vi "Programa funcion T co.vi"() -> ()   [LabVIEW 2020]
uses:
  <vilib>/addons/Control Design/_Model Construction/NI_LinSys_Model Creation.lvlib
  <vilib>/addons/Control Design/_Model Construction/NI_LinSys_Model Information.lvlib
  <vilib>/addons/Control Design/_Utility/NI_CD_Model Viewer.lvlib
  <vilib>/addons/Control Design/_Utility/Model Viewer.llb/Model Viewer SubVI/cd_Draw Transfer Function Equation (TF).vi
  <vilib>/addons/Control Design/_Model Construction/Model Information.llb/Model Information SubVIs/cd_Set Names To TF Model.vi
  <vilib>/addons/Control Design/_Model Construction/Model Creation.llb/Model Creation SubVI/cd_Create Transfer Function Model.vi
  <vilib>/functionblocks/Control/PID/PID.vi
  <vilib>/functionblocks/FB Core/FB Core.xnode
panel:
  out "?":T1(graph)={"Set-point (%)"=25.0, "Y% esc y filt"=25.0, "Ley uk"=12.500000564078626}
  in  "SET-POINT %":dbl
  in  "Ring":u16(ring) items=["LAZO ABIERTO", "LAZO CERRADO"]
  out "Y(k)":dbl
  out "X(t)":dbl[](array[numeric])
  in  "stop":bool
  in  "RETARDO":dbl
  in  "DENOMIDADOR":dbl[](array[numeric])
  in  "NUMERADOR":dbl[](array[numeric])
  out "Funcion de transferencia":picture
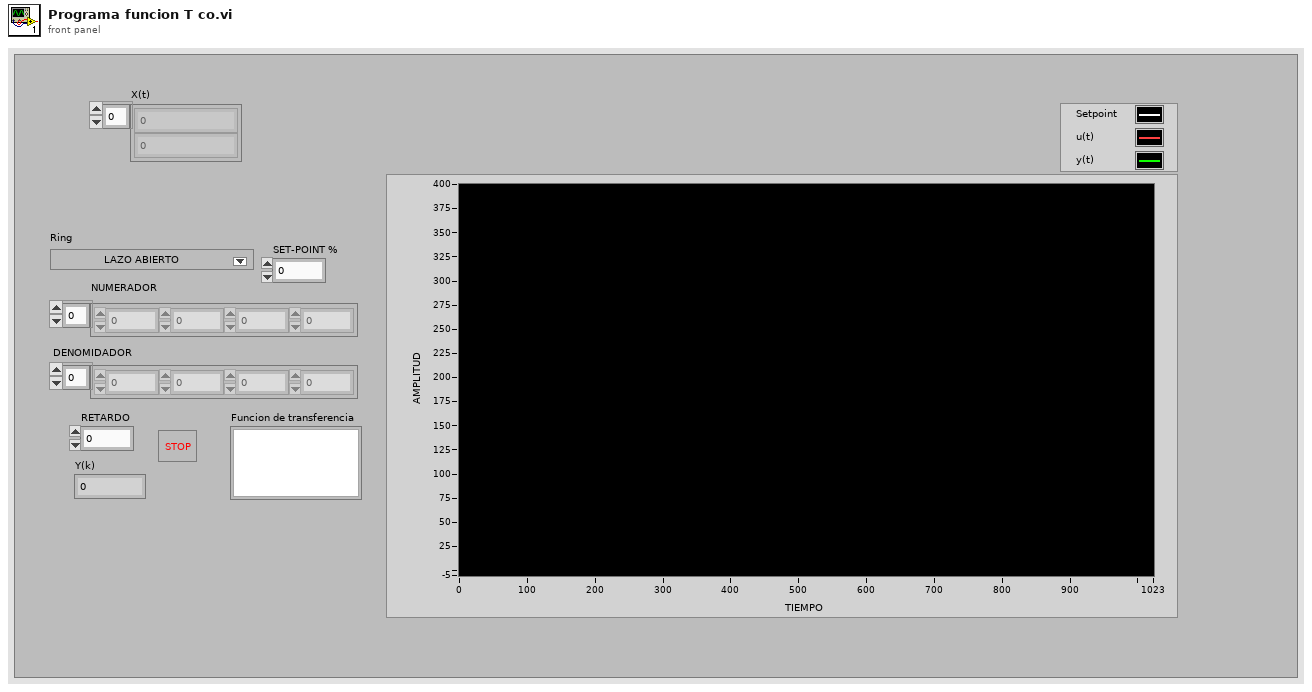
[diagram p1: front panel]
types:
  T1 = cluster{"Set-point (%)":dbl, "Y% esc y filt":dbl, "Ley uk":dbl}
  T2 = typedef "NI_Matrix.lvlib/RealMatrix.ctl" = dbl[][]
  T3 = cluster{"SET-POINT %":dbl, "output":dbl, "Y(k)":dbl}
  T4 = typedef "NI_LinSys_Model Typedefs.lvlib/CD Transfer Function Model (MIMO).ctl" = cluster{"properties":T5, "transfer function(s)":T6[][]}
  T5 = typedef "NI_LinSys_Model Typedefs.lvlib/CD General Elements.ctl" = cluster{"Model name":string, "Input names":string[], "Output names":string[], "Input Delays":dbl[], "Output Delays":dbl[], "Sampling Time":dbl, "Notes":string}
  T6 = typedef "NI_LinSys_Model Typedefs.lvlib/CD Transfer Function Model (SISO).ctl" = cluster{"Numerator":dbl[], "Denominator":dbl[], "delay":dbl}
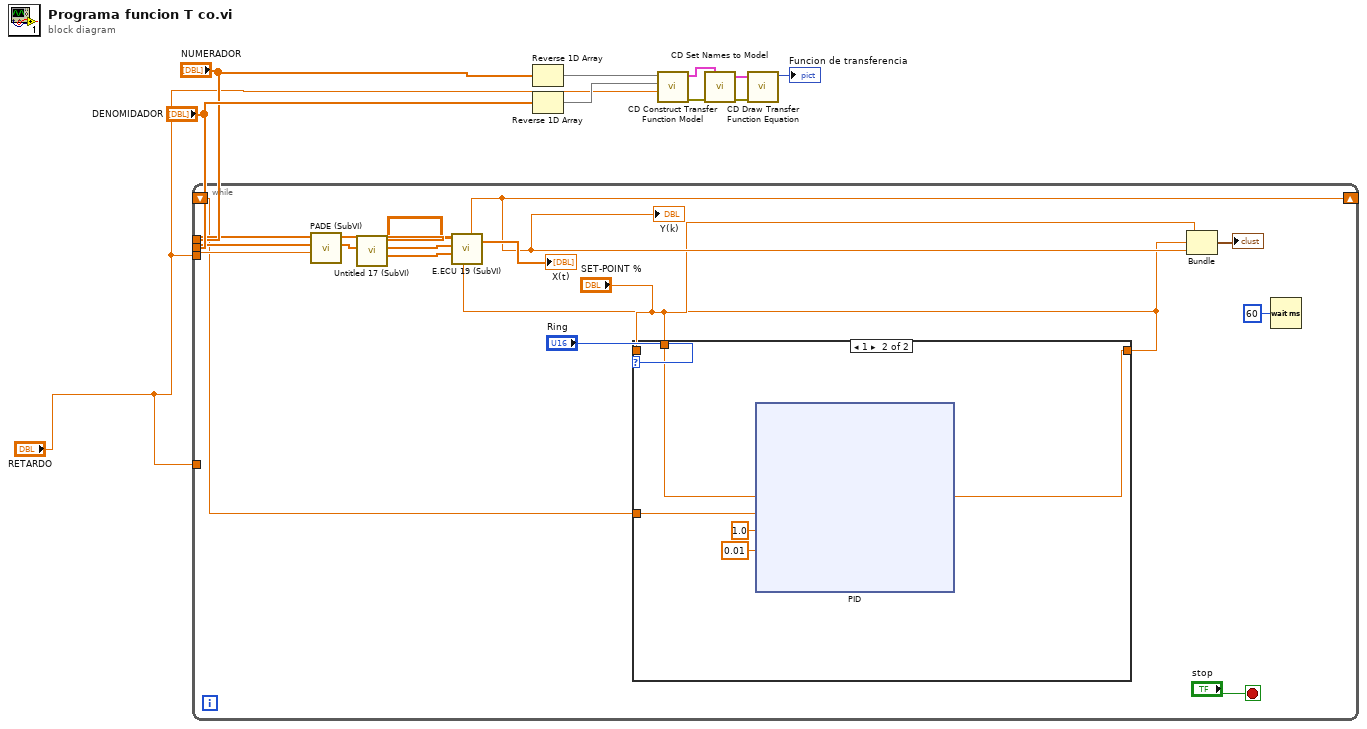
[diagram p0: block diagram]
diagram:
  n1 = while {
    tunnel: "DENOMIDADOR" -> [w16]
    tunnel: "NUMERADOR" -> [w17]
    tunnel: "RETARDO" -> [w27]
    shift-right: [w15] -> _
    shift-left: _ -> [w12]
    tunnel: "RETARDO" -> [_]
    stop <- "stop" stop-if-true
    n2 = call "PADE (SubVI).vi"("RETARDO"=w27, "DENOMIDADOR"=w16, "NUMERADOR"=w17) -> ("DENOMIDADOR  PADE"=w25:dbl[], "NUMERADOR  PADE"=w24:dbl[])  [unwired: 7 in]
    n3 = call "Untitled 17 (SubVI).vi"("DENOMIDADOR  PADE"=w25, "NUMERADOR  PADE"=w24) -> ("C"=w22:dbl[], "B"=w21:dbl[], "A"=w23:T2)  [unwired: 7 in]
    n4 = case shown="1" "Ring" {
      tunnel: "SET-POINT %" -> [w28 _]
      tunnel: [w28 w29] -> w11
      tunnel: "SET-POINT %" -> [_ w33]
      tunnel: w12 -> [_ w32]
      frame 0, Default {
      }
      frame 1 {
        n5 = xnode "PID"("setpoint"=w33, "process variable"=w32, "proportional gain (Kc)"=1.0, "integral time (Ti, min)"=0.01) -> ("output"=w29:dbl)  [unwired: 3 in, 1 out]
      }
    }
    n6 = call "E.ECU 19 (SubVI).vi"("u(k)"=w11, "C in"=w22, "B in"=w21, "A in"=w23) -> ("Y(k)"=w15:dbl, "X(t)"=→"X(t)":dbl[])  [unwired: 6 in]
    "Y(k)" <- w15
    n7 = Bundle("SET-POINT %"="SET-POINT %", "output"=w11, "Y(k)"=w15) -> (→"?":T3)  [unwired: 1 in]
    n8 = Wait (ms)(milliseconds to wait=u32 60) -> ()  [unwired: 1 out]
  }
  n9 = Reverse 1D Array(array="NUMERADOR") -> (reversed array=w5:dbl[])
  n10 = Reverse 1D Array(array="DENOMIDADOR") -> (reversed array=w4:dbl[])
  n11 = call-poly <vilib>:"CD Construct Transfer Function Model.vi"("Delay"="RETARDO", "Denominator"=w4, "Numerator"=w5) -> ("error out"=w8:errorcluster, "Transfer Function Model"=w6:T4)  [unwired: 7 in]
  n12 = call-poly <vilib>:"CD Set Names to Model.vi"("Transfer Function Model In"=w6, "error in (no error)"=w8) -> ("Model Out"=w7:T4, "error out"=w9:errorcluster)  [unwired: 12 in]
  n13 = call-poly <vilib>:"CD Draw Transfer Function Equation.vi"("error in (no error)"=w9, "Transfer Function Model"=w7) -> ("Equation"=→"Funcion de transferencia":picture)  [unwired: 7 in, 2 out]
